vi "GetInputtypes.vi"(0 "reference in":refnum<class "Executer.lvclass">, 1 "Class":string, 2 "Method":string, 5 "error in (no error)":errorcluster) -> (14 "reference out":refnum<class "Executer.lvclass">, 17 "InputTypes":variant[](array[variant]), 19 "error out":errorcluster)   [LabVIEW 2018, in "Executer.lvclass"]
uses:
  Executer.lvclass
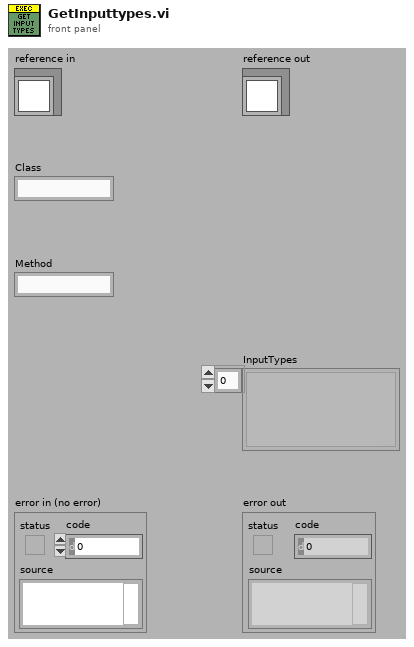
[diagram p1: front panel]
types:
  T1 = typedef "Executer.lvclass/MethodExecutionInfo.ctl" = cluster{"viRef":refnum<vi>, "MethodName":string, "ControlIndices":i32[], "ClassInIndex":i32, "IndicatorIndices":i32[], "ErrorOutIndex":i32, "ControlTypes":variant[]}
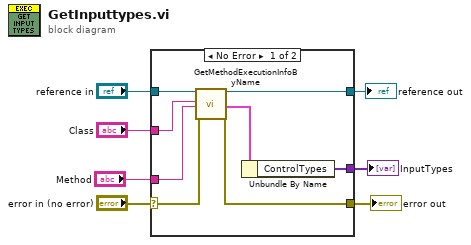
[diagram p0: block diagram]
diagram:
  n1 = case shown="No Error" "error in (no error)" {
    selector: "error in (no error)" -> [w15 w17]
    tunnel: [w9 w17] -> w6
    tunnel: [w13 w16] -> w4
    tunnel: "reference in" -> [w14 w16]
    tunnel: "Class" -> [w12 _]
    tunnel: "Method" -> [w11 _]
    tunnel: [w8 _] -> w1
    frame No Error {
      n2 = call "GetMethodExecutionInfoByName.vi"("Executer in"=w14, "Class in"=w12, "Method"=w11, "error in (no error)"=w15) -> ("Executer out"=w13:refnum<class "Executer.lvclass">, "Method"=w10:T1, "error out"=w9:errorcluster)  [unwired: 12 in, 1 out]
      n3 = Unbundle By Name(w10) -> ("ControlTypes"=w8:variant[])
    }
    frame Error {
    }
  }
  "error out" <- w6
  "reference out" <- w4
  "InputTypes" <- w1
